vi "simulation of servo has NO integrator.vi"() -> ()   [LabVIEW 2021]
uses:
  <vilib>/addons/Control Design/_Model Construction/Model Typedefs.llb/CD State Space Model (MIMO).ctl
  <vilib>/addons/Control Design/_Model Construction/Model Typedefs.llb/CD General Elements.ctl
  <vilib>/Analysis/Matrix/Datatypes/RealMatrix.ctl
  <vilib>/Simulation/Scripting/Companion Diagram/SimConfigNode/SimParams.ctl
  <vilib>/Simulation/Scripting/Companion Diagram/SimConfigNode/_simSolvers.ctl
  <vilib>/Simulation/Implementation/Shared/SIMSCR Execution Mode.ctl
  <vilib>/Simulation/Param Hierarchy/Typedefs/SIMPH Param Control Actions.ctl
  <vilib>/Simulation/Implementation/Shared/SIM limit type.ctl
  <vilib>/Simulation/Implementation/Shared/NILVSim_ParamChanged.vi
  <vilib>/Simulation/Implementation/Shared/NILVSIM_BeginStep.vi
  <vilib>/Simulation/DataSources/Implementation/NILVSim Step.llb/SIM Step (scalar).vi
  <vilib>/Simulation/ContinuousLinear/Implementation/NILVSim Integrator new.llb/SIM Integrator Distributor (vector).vi
  <vilib>/Simulation/SignalArithmetic/Implementation/NILVSim Gain.llb/SIM Gain (vector,ScalarGain).vi
  <vilib>/Simulation/ContinuousLinear/Implementation/NILVSim State Space.llb/SIM State Space Distributor (CD).vi
  <vilib>/Simulation/SignalArithmetic/Implementation/NILVSim Gain.llb/SIM Gain (vector,MatrixGain).vi
  <vilib>/Simulation/ContinuousLinear/Implementation/NILVSim State Space.llb/SIM State Space Collector (CD).vi
  <vilib>/Simulation/SignalDisplay/Implementation/NILVSim Time Waveform.llb/SIM Time Waveform (vector).vi
  <vilib>/Simulation/ContinuousLinear/Implementation/NILVSim Integrator new.llb/SIM Integrator Collector (vector).vi
  <vilib>/Simulation/Implementation/Shared/NILVSim_Manager.vi
  <vilib>/Utility/error.llb/Clear Errors.vi
  <vilib>/Simulation/Implementation/Shared/NILVSim_FinalizeModel.vi
  <vilib>/addons/Control Design/_Model Construction/Model Creation.llb/Model Creation SubVI/cd_Create State Space Model.vi
  <vilib>/addons/Control Design/_Dynamic Analysis/Dynamic Analysis.llb/Dynamic Analysis subVI/cd_Poles (State-Space).vi
  <vilib>/addons/Control Design/_Dynamic Analysis/Dynamic Analysis.llb/Dynamic Analysis subVI/cd_Pole-Zero Map (State-Space).vi
  <vilib>/addons/Control Design/_Utility/Model Viewer.llb/Model Viewer SubVI/cd_Draw State-Space Equation (SS).vi
  <vilib>/Analysis/baseanly.llb/Real Inverse Matrix.vi
  <vilib>/Simulation/Implementation/Shared/SIM Unbundle Sim Info.vi
  <vilib>/Simulation/Implementation/Shared/NILVSim_Initialize.vi
  <vilib>/Simulation/Utility/Implementation/NILVSim Get Time and IsAcceptedStep.vi
  <vilib>/Simulation/Implementation/Shared/SIMSH Read Queue.vi
  <vilib>/Simulation/Implementation/Shared/NILVSim_GetModelError.vi
  <vilib>/Simulation/Implementation/Shared/SIM Bundle Sim Info.vi
  <vilib>/Simulation/Scripting/Companion Diagram/SimConfigNode/SimDog.xnode
  <vilib>/Simulation/Implementation/XNodeFramework/SimXNode/SimX.xnode
  <vilib>/addons/Control Design/_Model Construction/NI_LinSys_Model Creation.lvlib
  <vilib>/addons/Control Design/_State-Space Analysis/NI_CD_State-Space Analysis.lvlib
  <vilib>/addons/Control Design/_Utility/NI_CD_Model Viewer.lvlib
  <vilib>/Analysis/NI_AALBase.lvlib
  <vilib>/addons/Control Design/_State Feedback Control/NI_CD_State Feedback Control.lvlib
  <vilib>/addons/Control Design/_Dynamic Analysis/NI_CD_Dynamic Analysis.lvlib
  <vilib>/addons/Control Design/_Model Construction/NI_LinSys_Model Typedefs.lvlib
  <vilib>/Simulation/ContinuousLinear/Implementation/NILVSim State Space.llb/SIM State Space (CD).vi
  <vilib>/Simulation/ContinuousLinear/Implementation/NILVSim Integrator new.llb/SIM Integrator (vector).vi
  <vilib>/Simulation/Implementation/Shared/NI_SIM_Implementation.lvlib
  <vilib>/Analysis/Matrix/NI_Matrix.lvlib
panel:
  out "main k size)":i32[](array[numeric])
  out "[K1 K2 K3 K4 ....0]":dbl[][](array[numeric])
  out "Ki":dbl
  out "Waveform Chart":waveform(dbl)[](graph)
  in  "r(t)":dbl=1.0
  out "Open Loop Poles":cdb[](array[numeric])=[-1.0+0.0i, -2.0+0.0i] format="%.3f"
  out "K (Gain)":dbl[][](array[numeric])=[[6.500000000000002, 2.5000000000000004]] format="%.2f"
  in  "Gain Type":u16(ring) items=["Controller Gain", "Observer Gain (Predictive)", "Observer Gain (Current)"]
  in  "Desired Poles":cdb[](array[numeric])=[-3.0+0.0i, -5.0+0.0i] format="%.2f"
  out "Transformation Matrix(T)":T1=[[2.0, 0.0], [0.0, 2.0]]
  out "Equation":picture
  in  "Form Type":u16(ring)=1 items=["Modal"=0, "Companion"=5, "Controllability"=1, "Controller Companion"=2, "Observability"=3, "Observer Companion"=4]
  out "Transformation Matrix inverse (T')":dbl[][](array[numeric])=[[0.5, 0.0], [-0.0, 0.5]] format="%.2f"
  out "new Transformed Model":T2={"properties"={"Model name"="System Model", "Input names"=["u0"], "Output names"=["y0"], "Input Delays"=[0.0], "Output Delays"=[0.0], "Sampling Time"=0.0, "Notes"=""}, "A"=[[0.0, 1.0], [-2.0, -3.0]], "B"=[[0.0], [1.0]], "C"=[[2.0, 0.0]], "D"=[[0.0]], "StateNames"=["x0", "x1"], "Transport Delay"=[[0.0]]} {"Transport Delay" format="%.2f"; "D" format="%#.2g"; "C" format="%#.2g"; "B" format="%#.2g"; "A" format="%#.2g"; "properties"."Sampling Time" format="%#.6p"; "properties"."Output Delays" format="%.4f"; "properties"."Input Delays" format="%.4f"}
  out "Is Controllable?":bool=TRUE
  out "Controllability Matrix (M)":dbl[][](array[numeric])=[[0.0, 2.0], [2.0, -6.0]] format="%.2f"
  in  "D":dbl[][](array[numeric])=[[0.0]] format="%#.5g"
  in  "C":dbl[][](array[numeric])=[[1.0, 0.0]] format="%#.5g"
  in  "B":dbl[][](array[numeric])=[[0.0], [2.0]] format="%#.5g"
  in  "A":dbl[][](array[numeric])=[[0.0, 1.0], [-2.0, -3.0]] format="%#.5g"
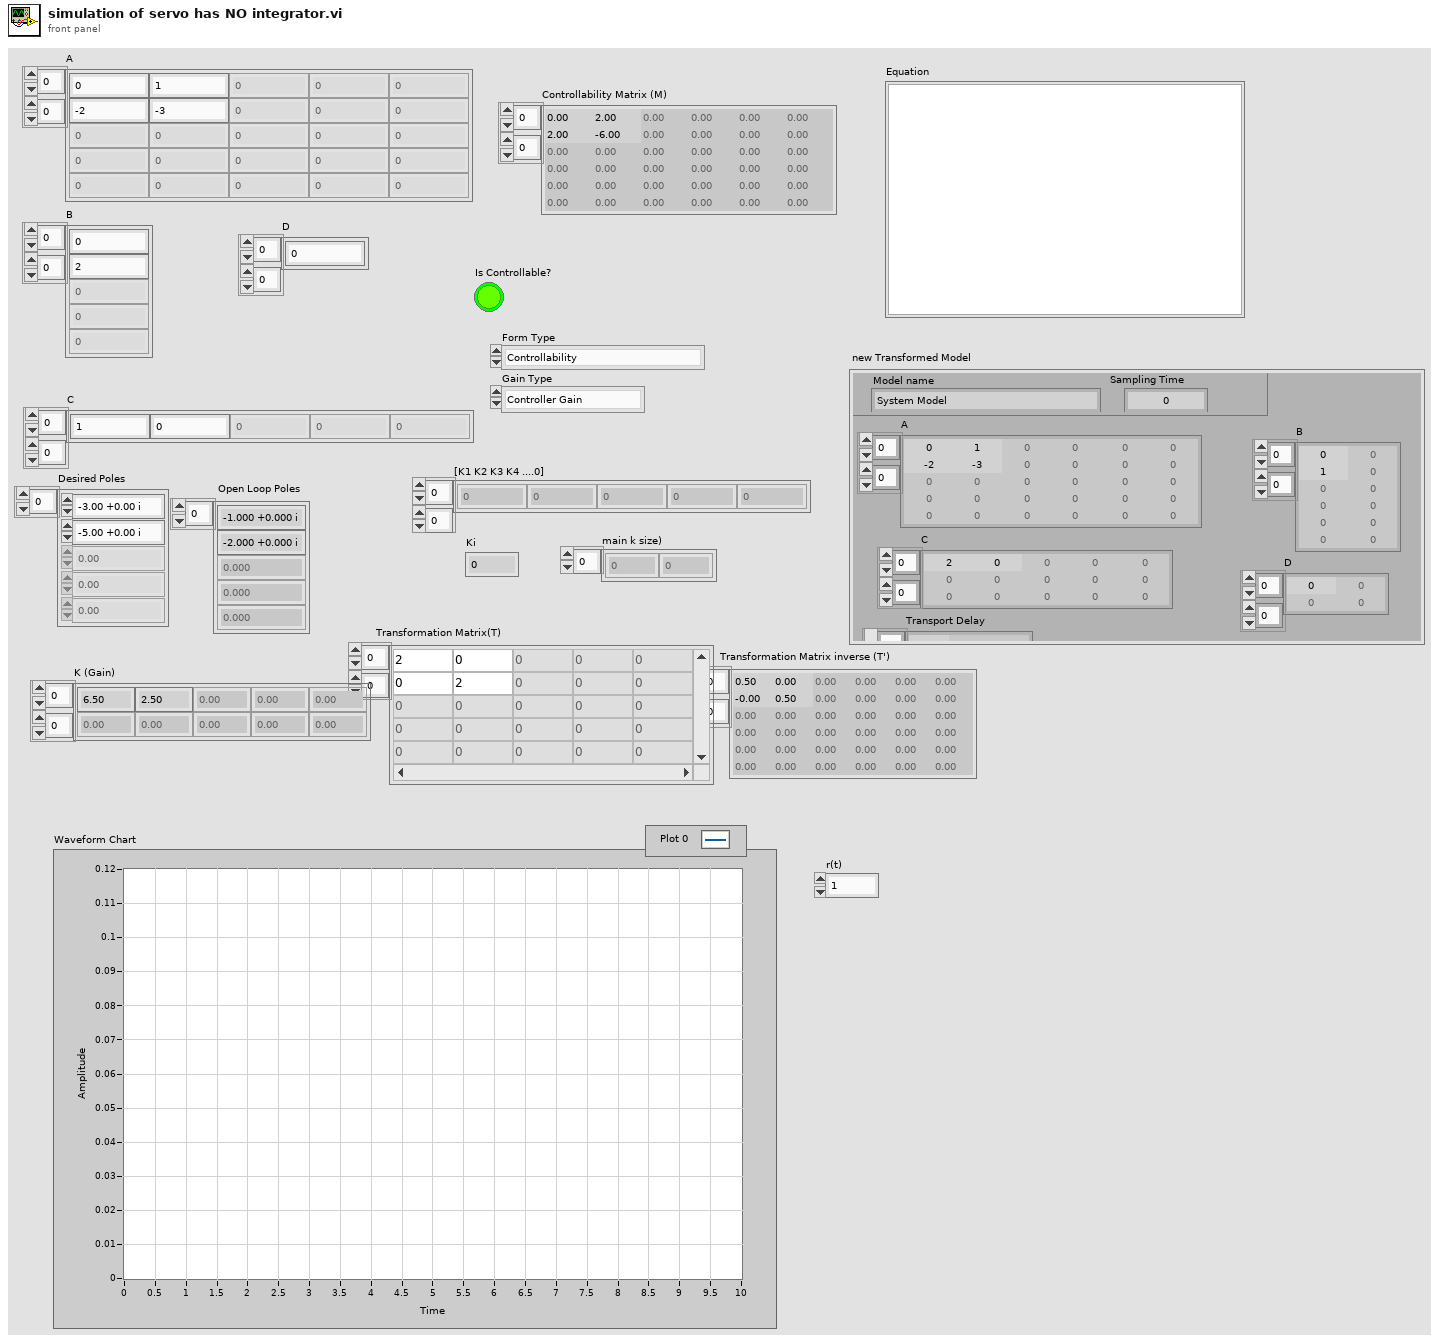
[diagram p1: front panel]
types:
  T1 = typedef "NI_Matrix.lvlib/RealMatrix.ctl" = dbl[][]
  T2 = typedef "NI_LinSys_Model Typedefs.lvlib/CD State Space Model (MIMO).ctl" = cluster{"properties":T3, "A":dbl[][], "B":dbl[][], "C":dbl[][], "D":dbl[][], "StateNames":string[], "Transport Delay":dbl[][]}
  T3 = typedef "NI_LinSys_Model Typedefs.lvlib/CD General Elements.ctl" = cluster{"Model name":string, "Input names":string[], "Output names":string[], "Input Delays":dbl[], "Output Delays":dbl[], "Sampling Time":dbl, "Notes":string}
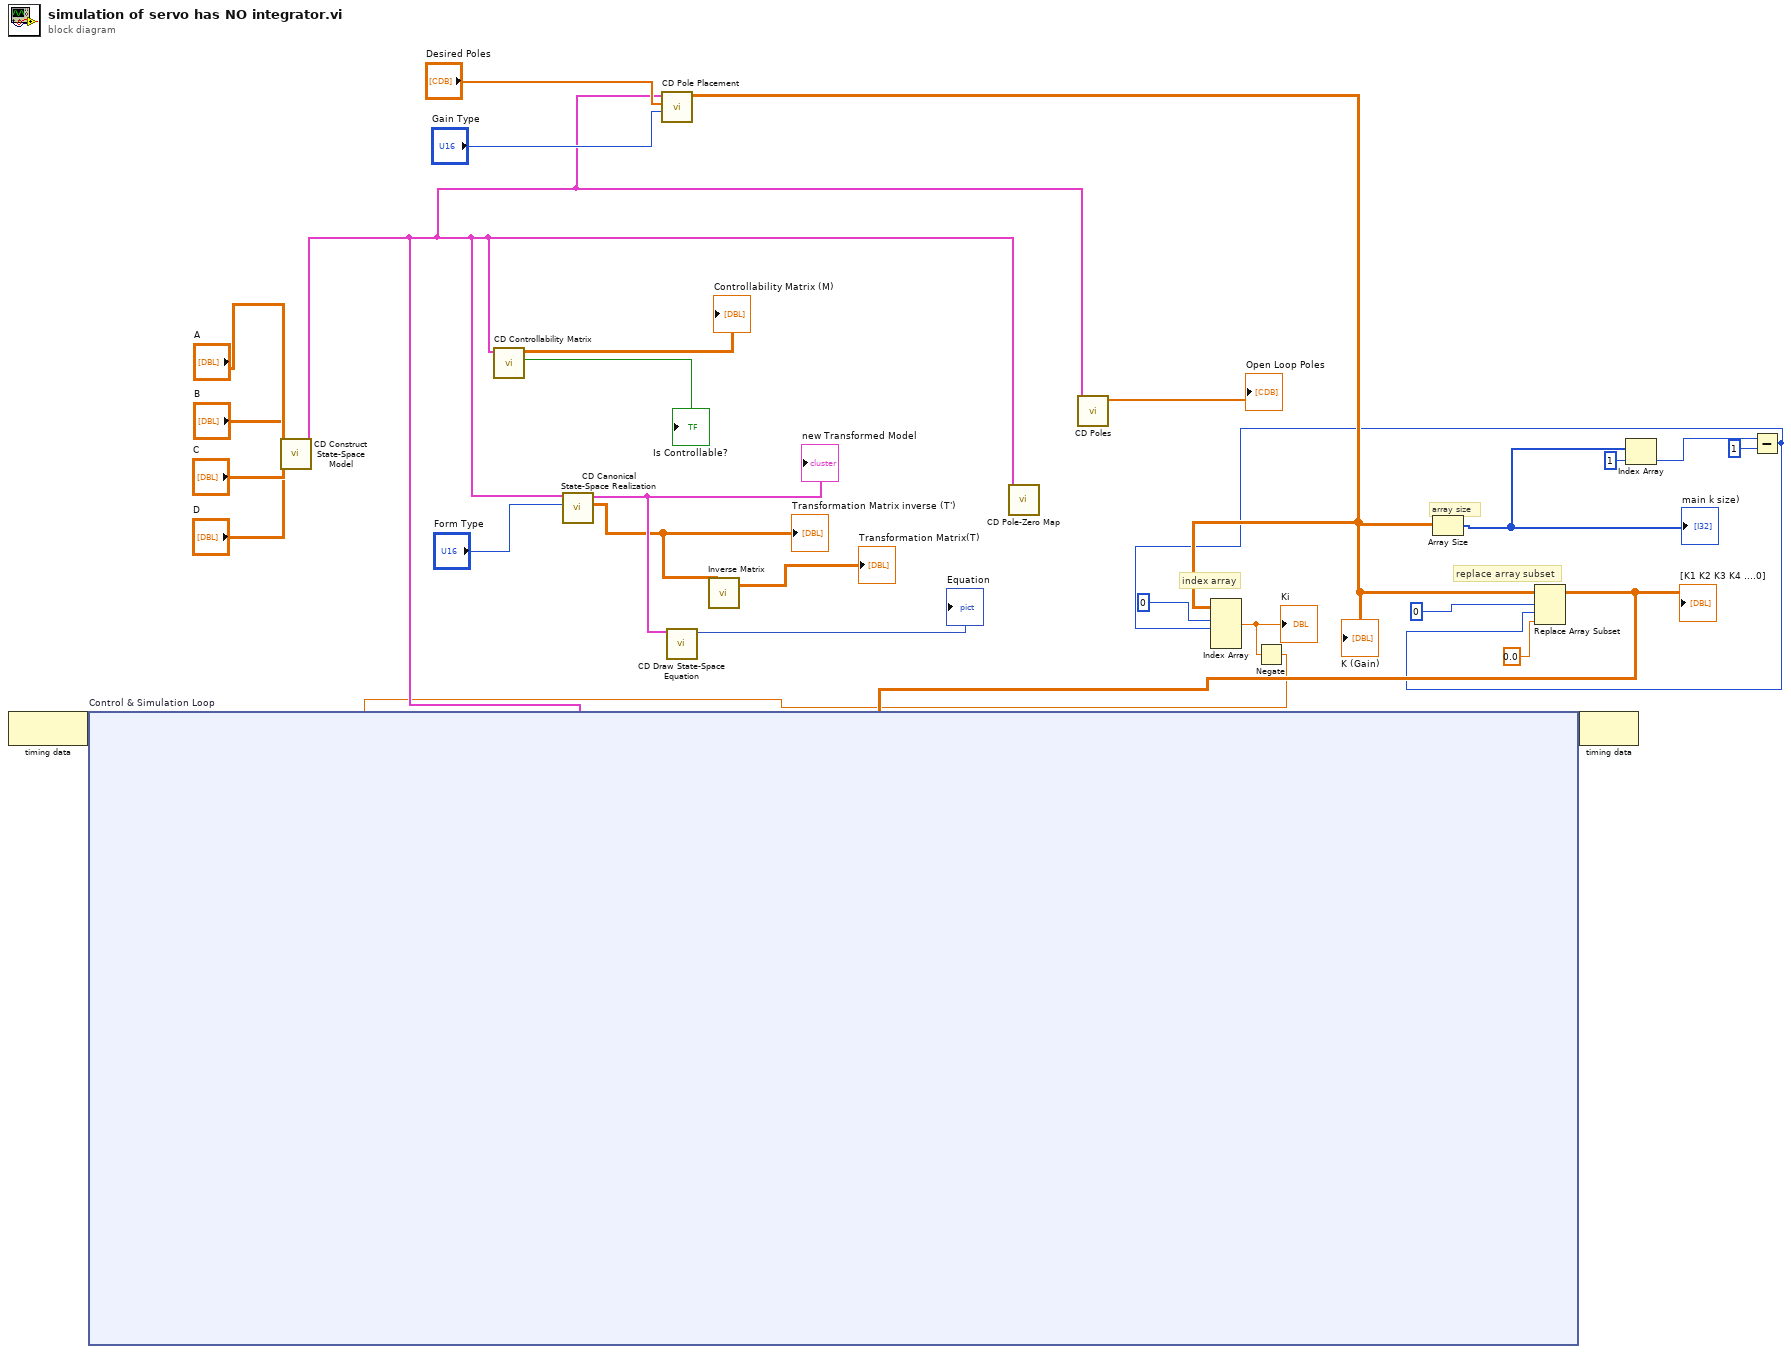
[diagram p0: block diagram]
diagram:
  # "array size"
  # "index array"
  # "replace array subset"
  n1 = node-c288() -> (w29:variant)  [unwired: 1 in]
  n2 = call-poly <vilib>:"CD Construct State-Space Model.vi"("A"="A", "B"="B", "C"="C", "D"="D") -> ("State-Space Model"=w13:T2)  [unwired: 10 in, 1 out]
  n3 = call <vilib>:"CD Controllability Matrix.vi"("State-Space Model"=w13) -> ("Is Controllable?"=→"Is Controllable?":bool, "Controllability Matrix"=→"Controllability Matrix (M)":dbl[][])  [unwired: 7 in, 2 out]
  n4 = call <vilib>:"CD Canonical State-Space Realization.vi"("Form Type"="Form Type", "State-Space Model"=w13) -> ("Transformation Matrix (T)"=w22:dbl[][], "Transformed Model"=w24:T2)  [unwired: 7 in, 1 out]
  "new Transformed Model" <- w24
  "Transformation Matrix inverse (T')" <- w22
  n5 = call <vilib>:"CD Pole Placement.vi"("Gain Type"="Gain Type", "Poles"="Desired Poles", "State-Space Model"=w13) -> ("Gain"=w8:dbl[][])  [unwired: 6 in, 2 out]
  "K (Gain)" <- w8
  n6 = call-poly <vilib>:"CD Draw State-Space Equation.vi"("State-Space Model"=w24) -> ("Equation"=→"Equation":picture)  [unwired: 8 in, 2 out]
  n7 = call-poly <vilib>:"Inverse Matrix.vi"("Input Matrix"=w22) -> ("Inverse Matrix"=→"Transformation Matrix(T)":T1)  [unwired: 1 in, 1 out]
  n8 = call-poly <vilib>:"CD Pole-Zero Map.vi"("State-Space Model"=w13) -> ()  [unwired: 7 in, 4 out]
  n9 = call-poly <vilib>:"CD Poles.vi"("State-Space Model"=w13) -> ("Poles"=→"Open Loop Poles":cdb[])  [unwired: 9 in, 1 out]
  n10 = Array Size(array=w8) -> (size(s)=w7:i32[])
  "main k size)" <- w7
  n11 = Index Array(array=w7, index=1) -> (element=w5:i32)
  n12 = Subtract(x=w5, y=1) -> (x-y=w3:i32)
  n13 = Index Array(array=w8, index (row) #1=0 ("index (row)"), index (col) #1=w3) -> (element #1=w2:dbl)  [unwired: 2 in, 1 out]
  "Ki" <- w2
  n14 = Negate(x=w2) -> (-x=w1:dbl)
  n15 = Replace Array Subset(array=w8, new element=0.0 ("new element/subarray"), index (row)=0, index (col)=w3) -> (w9:dbl[][])
  "[K1 K2 K3 K4 ....0]" <- w9
  n16 = node-c254 "Control & Simulation Loop"(w29, w13, w1, w9) -> (w28:variant)
  n17 = node-c288(w28) -> ()  [unwired: 1 out]
